vi "PH_BeamlineController.set current Value of PA DP Target Elements.vi"(0 "VI in":refnum<vi>, 5 "error in (no error)":errorcluster) -> (14 "VI out":refnum<vi>, 19 "error out":errorcluster)   [LabVIEW 2014, in "PH_BeamlineController.lvlib"]
uses:
  PH_BeamlineController.lvlib
  PH_Beamline_Chief/PH_Beamline_Chief.Section.ctl
  PH_BeamlineInformation/PH_BeamlineInformation.lvlib
  PH_Beamline_Chief/PH_Beamline_Chief.lvlib
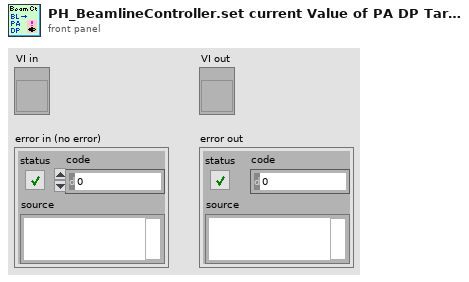
[diagram p1: front panel]
types:
  T1 = typedef "PH_BeamlineController.lvlib/PH_BeamlineController.i attribute.ctl" = cluster{"Vacuum Exp LB":cluster{"Channel":string, "Limit [mbar]":dbl, "Pressure [mbar]":dbl, "GUI Ref":refnum<vi>}, "Sources":T2[], "PA DP Targets":T4[], "Path":cluster{"Source":T3, "PA DP Target":T5, "Target":T6}, "Targets":cluster{"Name":T6, "GUI Ref":refnum<vi>, "Current State":bool, "Wanted State":bool, "Enabled":bool}[], "Status Tags":cluster{"Name":string, "Status":T7}[], "special GUI Refs":T8}
  T2 = typedef "PH_BeamlineController.lvlib/PH_BeamlineController.Source Attributes.ctl" = cluster{"Name":T3, "GUI Ref":refnum<vi>, "Current State":bool, "Wanted State":bool}
  T3 = typedef "PH_BeamlineController.lvlib/PH_BeamlineController.Sources.ctl" = enum16{"None", "YLF", "fs-Frontend", "ns-Frontend", "YLF and ns-Frontend", "fs- and ns-Frontend"}
  T4 = typedef "PH_BeamlineController.lvlib/PH_BeamlineController.PA DP Target Attributes.ctl" = cluster{"Name":T5, "GUI Ref":refnum<vi>, "Current State":bool, "Wanted State":bool, "Enabled":bool}
  T5 = typedef "PH_BeamlineController.lvlib/PH_BeamlineController.PA DP Targets.ctl" = enum16{"None", "Dump PA Delayed Beam", "Dump PA Undelayed Beam", "Dumps PA Delayed and Undelayed Beam"}
  T6 = typedef "PH_BeamlineController.lvlib/PH_BeamlineController.Targets.ctl" = enum16{"None", "PreAmp", "Dump Exp Laserlab", "Exp Laserlab", "Calorimeter", "Dump Exp Laserbay", "Exp Laserbay", "Dump Exp Z6", "Exp Z6"}
  T7 = typedef "PH_StatusHandler.lvlib/PH_StatusHandler.Status.ctl" = i16
  T8 = typedef "PH_BeamlineController.lvlib/PH_BeamlineController.special GUI Refs.ctl" = cluster{"PA-Backreflection-Meas":refnum<vi>, "fs_Synchrolock_Watch":refnum<vi>}
  T9 = typedef "PH_Beamline_Chief.lvlib/PH_Beamline_Chief.Section.ctl" = enum16{"None", "YLF", "fs", "fs-YLF", "ns", "PA-Input", "PA-Undelay", "PA-Delay", "PA-before-Bypass", "PA", "PA-Bypass", "PA-Exit", "PA-LL", "LL", "PA-MA", "MA-Exit", "MA-Z6", "Z6", "MA-LB", "LB-TB2", "LB-TB3"}
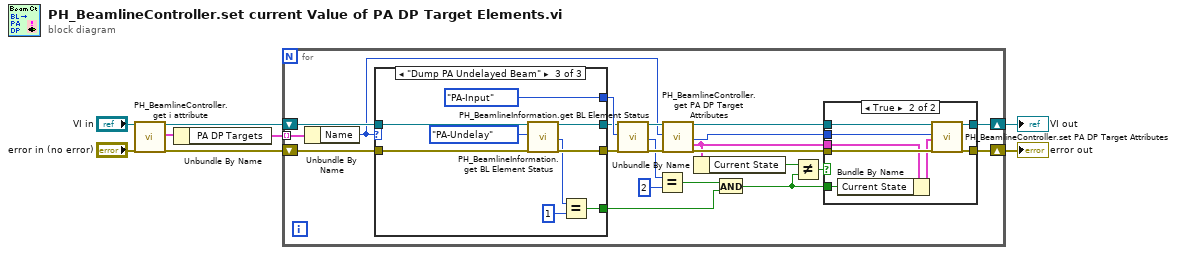
[diagram p0: block diagram]
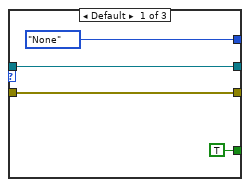
[diagram p2: hidden frame]
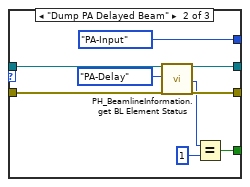
[diagram p3: hidden frame]
diagram:
  n1 = call "PH_BeamlineController.get i attribute.vi"("i ref in"="VI in", "error in (no error)"="error in (no error)") -> ("i ref out"=w4:refnum<vi>, "i attribute"=w8:T1, "error out"=w3:errorcluster)  [unwired: 15 in]
  n2 = Unbundle By Name(w8) -> ("PA DP Targets"=w5:T4[])
  n3 = for {
    shift-right: [w29] -> w7
    shift-left: w3 -> [w13]
    shift-right: [w27] -> w6
    shift-left: w4 -> [w15]
    tunnel: w5 -> [w25] mode=indexing
    n4 = Unbundle By Name(w25) -> ("Name"=w9:T5)
    n5 = case shown="\"Dump PA Undelayed Beam\"" w9 {
      tunnel: [PH_Beamline_Chief.Section."None" ("Beamline Element") PH_Beamline_Chief.Section."PA-Input" ("Beamline Element") PH_Beamline_Chief.Section."PA-Input" ("Beamline Element")] -> w19
      tunnel: w15 -> [w33 w40 w49]
      tunnel: [w33 w39 w48] -> w14
      tunnel: w13 -> [w32 w42 w51]
      tunnel: [w32 w41 w50] -> w12
      tunnel: [TRUE w35 w44] -> w10
      frame Default {
      }
      frame "Dump PA Delayed Beam" {
        n6 = call "PH_BeamlineInformation.get BL Element Status.vi"("VI in"=w40, "Beamline Element"=PH_Beamline_Chief.Section."PA-Delay", "error in (no error)"=w42) -> ("VI out"=w39:refnum<vi>, "Status"=w36:i32, "error out"=w41:errorcluster)  [unwired: 14 in]
        n7 = Equal?(x=w36, y=1) -> (x = y?=w35:bool)
      }
      frame "Dump PA Undelayed Beam" {
        n8 = call "PH_BeamlineInformation.get BL Element Status.vi"("VI in"=w49, "Beamline Element"=PH_Beamline_Chief.Section."PA-Undelay", "error in (no error)"=w51) -> ("VI out"=w48:refnum<vi>, "Status"=w45:i32, "error out"=w50:errorcluster)  [unwired: 14 in]
        n9 = Equal?(x=w45, y=1) -> (x = y?=w44:bool)
      }
    }
    n10 = call "PH_BeamlineInformation.get BL Element Status.vi"("VI in"=w14, "Beamline Element"=w19, "error in (no error)"=w12) -> ("VI out"=w21:refnum<vi>, "Status"=w18:i32, "error out"=w20:errorcluster)  [unwired: 14 in]
    n11 = Equal?(x=w18, y=2) -> (x = y?=w16:bool)
    n12 = call "PH_BeamlineController.get PA DP Target Attributes.vi"("VI in"=w21, "PA DP Target"=w9, "error in (no error)"=w20) -> ("VI out"=w28:refnum<vi>, "PA DP Target Index"=w26:i32, "PA DP Target Attributes"=w24:T4, "error out"=w30:errorcluster)  [unwired: 13 in]
    n13 = Unbundle By Name(w24) -> ("Current State"=w23:bool)
    n14 = And(x=w16, y=w10) -> (x .and. y?=w11:bool)
    n15 = Not Equal?(x=w23, y=w11) -> (x != y?=w22:bool)
    n16 = case shown="True" w22 {
      tunnel: w30 -> [w53 w62]
      tunnel: [w53 w61] -> w29
      tunnel: w28 -> [w54 w60]
      tunnel: [w54 w59] -> w27
      tunnel: w26 -> [_ w58]
      tunnel: w24 -> [_ w56]
      tunnel: w11 -> [_ w55]
      frame False {
      }
      frame True {
        n17 = Bundle By Name(cluster=w56, "Current State"=w55) -> (w57:T4)
        n18 = call "PH_BeamlineController.set PA DP Target Attributes.vi"("VI in"=w60, "PA DP Target Index"=w58, "Changed PA DP Target Attributes"=w57, "error in (no error)"=w62) -> ("VI out"=w59:refnum<vi>, "error out"=w61:errorcluster)  [unwired: 14 in]
      }
    }
  }
  "VI out" <- w6
  "error out" <- w7
